vi "Teleop.vi"(10 "Match Info":T1={"Autonomous Elapsed Seconds"=0.0, "TeleOp Elapsed Seconds"=0.0, "Disabled Elapsed Seconds"=0.0, "Visited Autonomous"=FALSE, "Visited TeleOp"=FALSE, "Visited Disabled"=FALSE, "Autonomous Settings"={"Autonomous Style"=enum."Independent", "VI Refnum"=refnum}}, 11 "Call Context":T2) -> ()   [LabVIEW 2020]
doc: "This VI is called for each enabled TeleOp packet received from the DS. It is typically used to read from joysticks and other inputs and update I/O or setpoints for timed control loops. It should complete and return within 20 milliseconds or risk missing DS packets."
uses:
  <vilib>/Rock Robotics/WPI/DriverStation/WPI_DriverStationDerivedRobotMode.ctl
  <vilib>/Rock Robotics/WPI/DriverStation/WPI_DriverStationMatch Info.ctl
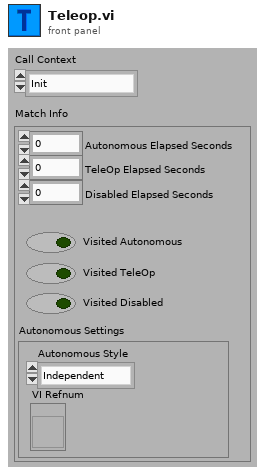
[diagram p1: front panel]
types:
  T1 = typedef "WPI_DriverStationMatch Info.ctl" = cluster{"Autonomous Elapsed Seconds":dbl, "TeleOp Elapsed Seconds":dbl, "Disabled Elapsed Seconds":dbl, "Visited Autonomous":bool, "Visited TeleOp":bool, "Visited Disabled":bool, "Autonomous Settings":cluster{"Autonomous Style":enum16{"Iterative", "Independent"}, "VI Refnum":refnum<vi>}}
  T2 = typedef "WPI_DriverStationDerivedRobotMode.ctl" = enum16{"Init", "Execute", "Stop"}
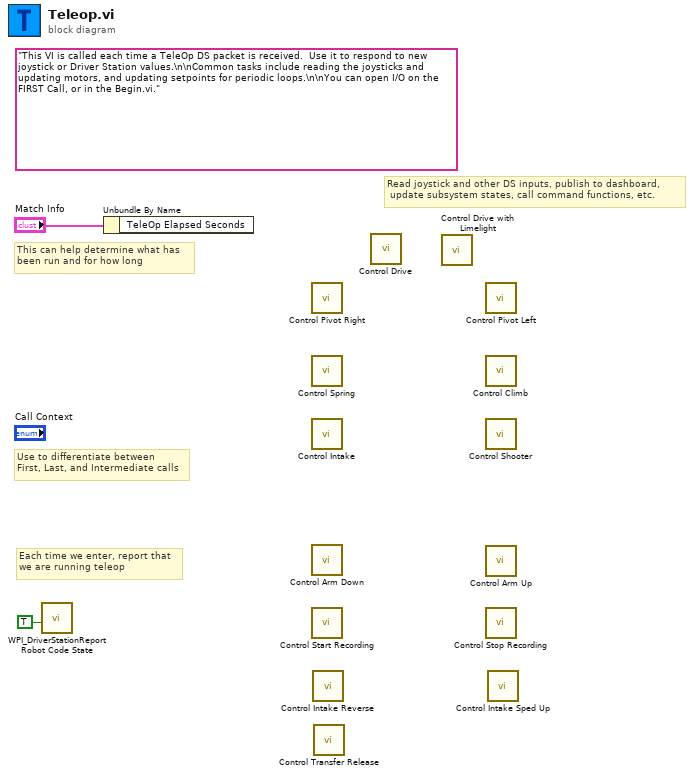
[diagram p0: block diagram]
diagram:
  (unwired) "This VI is called each time a TeleOp DS packet is received.  Use it to respond to new joystick or Driver Station values.\n\nCommon tasks include reading the joysticks and updating motors, and updating setpoints for periodic loops.\n\nYou can open I/O on the FIRST Call, or in the Begin.vi."
  # "Read joystick and other DS inputs, publish to dashboard,\n update subsystem states, call command functions, etc."
  # "Each time we enter, report that\nwe are running teleop"
  # "Use to differentiate between\nFirst, Last, and Intermediate calls"
  # "This can help determine what has\nbeen run and for how long"
  n1 = call <vilib>:"WPI_DriverStationReport Robot Code State.vi"("TeleOp"=TRUE ("Autonomous")) -> ()  [unwired: 10 in, 1 out]
  n2 = Unbundle By Name("Match Info") -> ()  [unwired: 1 out]
  n3 = call "Control Pivot Right.vi"() -> ()  [unwired: 12 in]
  n4 = call "Control Spring.vi"() -> ()  [unwired: 12 in]
  n5 = call "Control Intake.vi"() -> ()  [unwired: 12 in]
  n6 = call "Control Arm Down.vi"() -> ()  [unwired: 12 in]
  n7 = call "Control Start Recording.vi"() -> ()  [unwired: 12 in]
  n8 = call "Control Intake Reverse.vi"() -> ()  [unwired: 12 in]
  n9 = call "Control Transfer Release.vi"() -> ()  [unwired: 12 in]
  n10 = call "Control Drive.vi"() -> ()  [unwired: 12 in]
  n11 = call "Control Drive with Limelight.vi"() -> ()  [unwired: 12 in]
  n12 = call "Control Pivot Left.vi"() -> ()  [unwired: 12 in]
  n13 = call "Control Climb.vi"() -> ()  [unwired: 12 in]
  n14 = call "Control Shooter.vi"() -> ()  [unwired: 12 in]
  n15 = call "Control Arm Up.vi"() -> ()  [unwired: 12 in]
  n16 = call "Control Stop Recording.vi"() -> ()  [unwired: 12 in]
  n17 = call "Control Intake Sped Up.vi"() -> ()  [unwired: 12 in]
